vi "ReadNet_ModelOptimizer.vi"(8 "error in":errorcluster, 10 "Bin":path, 11 "Xml":path) -> (0 "error out":errorcluster, 3 "NET":refnum<class "NET.lvclass">)   [LabVIEW 2020, in "OpenLvVision_OpenCv.lvlib"]
doc: "Load a network from Intel's Model Optimizer intermediate representation."
uses:
  OpenLvVision_OpenCv.lvlib
  NET/NET.lvclass
  _LvHelpers/EdvrObject/TypeDef/Edvr.ctl
  _LvHelpers/EdvrObject/EdvrObject.lvclass
  Dlls/OlvOpenCvWrapper.dll
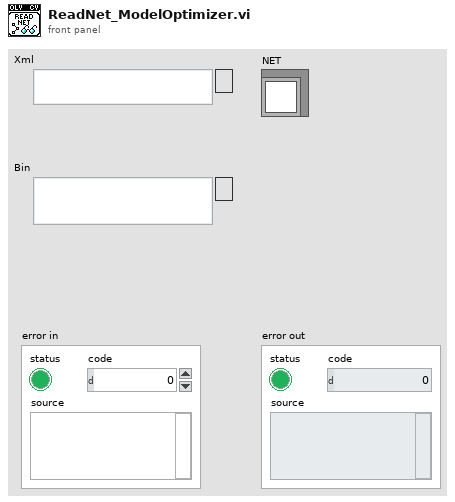
[diagram p1: front panel]
types:
  T1 = typedef "OpenLvVision_OpenCv.lvlib/EdvrObject.lvclass/Edvr.ctl" = refnum<data-value>
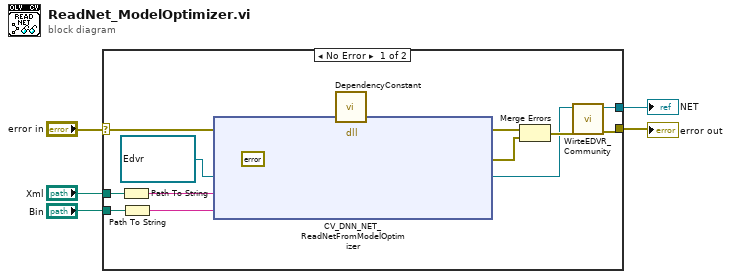
[diagram p0: block diagram]
diagram:
  n1 = case shown="No Error" "error in" {
    selector: "error in" -> [w16 w19]
    tunnel: [w14 w19] -> w4
    tunnel: [w12 _] -> w3
    tunnel: "Xml" -> [w11 _]
    tunnel: "Bin" -> [w9 _]
    frame No Error {
      n2 = Path To String(path=w11) -> (string=w10:string)
      n3 = Path To String(path=w9) -> (string=w8:string)
      n4 = dll-call lib="C:/Users/lukas/Downloads/OpenLvVision_OpenCv/SourceCode/LabView/OpenLvVision_OpenCv/Dlls/OlvOpenCvWrapper.dll" fn="CV_DNN_NET_ReadNetFromModelOptimizer"(error in=w16, "Error"=errorcluster {"status"=FALSE, "code"=0, "source"=""} ("error out"), "Edvr"=T1 refnum, "xml"=w10, "bin"=w8) -> (error out=w18:errorcluster, "Error"=w7:errorcluster, "Edvr"=w13:T1)  [unwired: 5 in, 1 out]
      n5 = call "DependencyConstant.vi"() -> ()  [unwired: 12 in]
      n6 = Merge Errors(w18, w7) -> (w15:errorcluster)
      n7 = call "WirteEDVR_Community.vi"("error in"=w15, "Edvr"=w13) -> ("error out"=w14:errorcluster, "NET"=w12:refnum<class "NET.lvclass">)  [unwired: 8 in]
    }
    frame Error {
    }
  }
  "NET" <- w3
  "error out" <- w4
